vi "main.vi"() -> ()   [LabVIEW 2018]
uses:
  State Enum.ctl
panel:
  in  "Acquisition time":dbl=1.0 caption="Time Target (s)" step=600.0 format="%<%H:%M:%S>t"
  out "Elapsed Time":dbl caption="Elapsed Time (s)" format="%<%H:%M:%S>t"
  in  "Stop":bool
  in  "Time between measurements":dbl=1.0 caption="Time Target (s)" step=10.0 format="%<%H:%M:%S>t"
  out "O3 Reading / V":dbl
  out "O3 Mean / V":dbl format="%0.2f"
  out "NOy Reading / V":dbl
  out "NOy Mean / V":dbl format="%0.2f"
  out "NO2 Reading / V":dbl
  out "NO2 Mean / V":dbl format="%0.2f"
  out "CRDS Voltage":dynamicdata(graph)
  out "NO Reading / V":dbl
  out "NO Mean / V":dbl format="%0.2f"
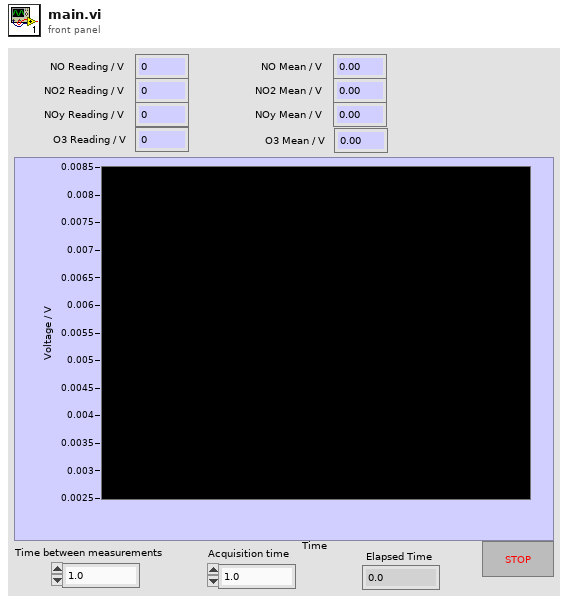
[diagram p1: front panel]
types:
  T1 = enum16{"Always On", "Always Off", "Off While Running"}
  T2 = typedef "State Enum.ctl" = enum16{"Acquisition", "Analysis", "Data Log", "Time Check"}
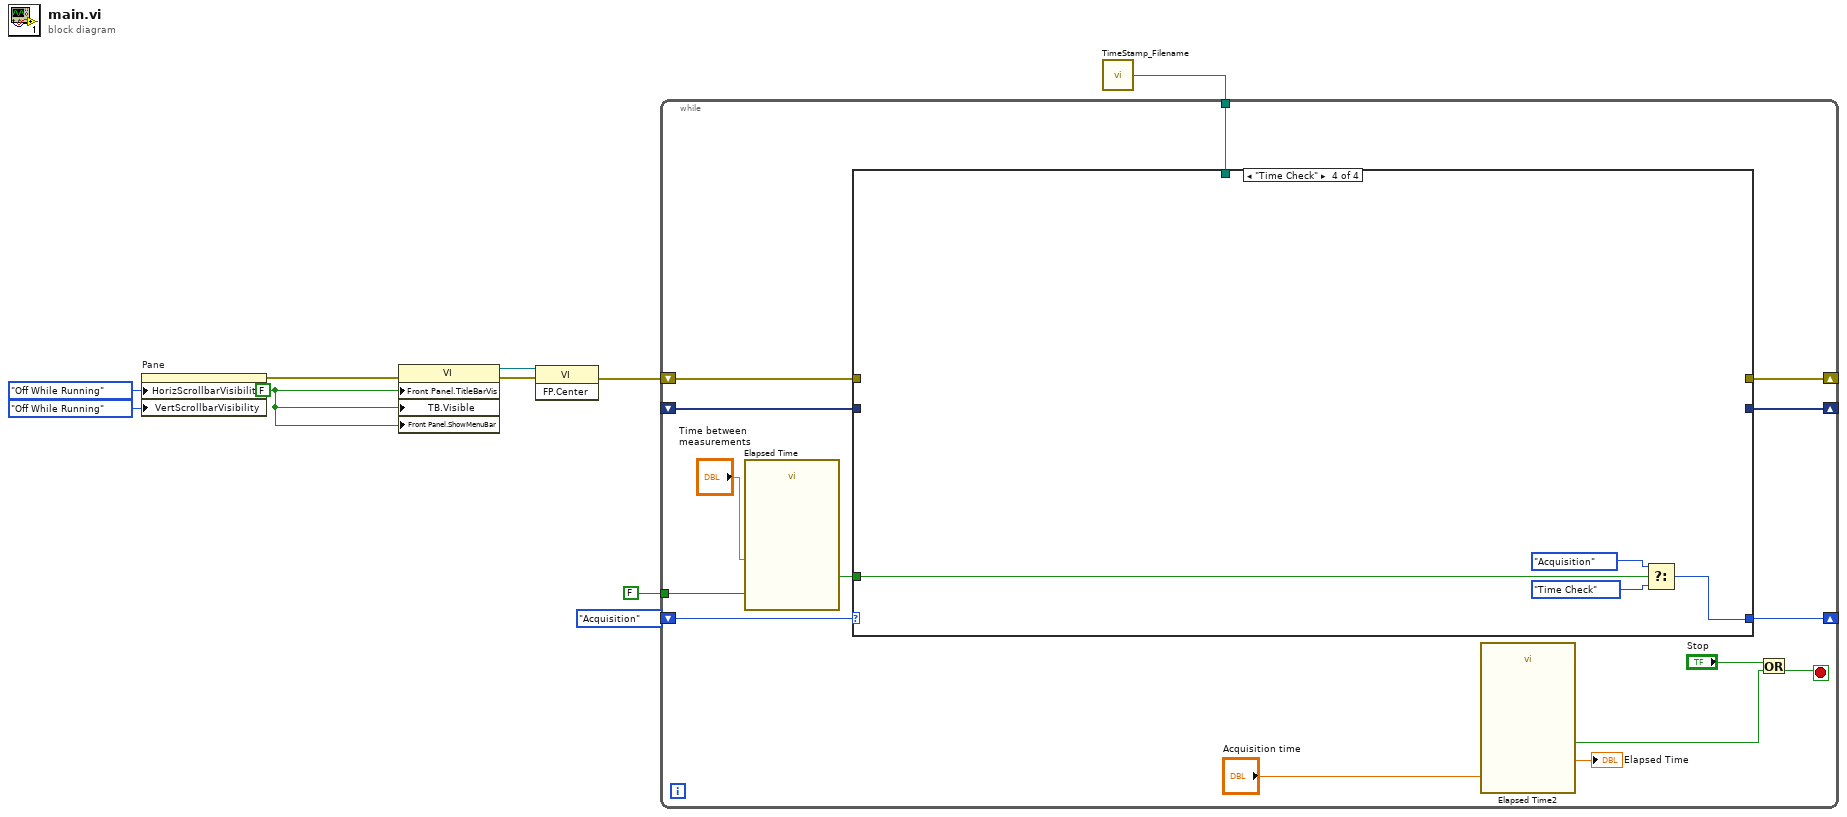
[diagram p0: block diagram]
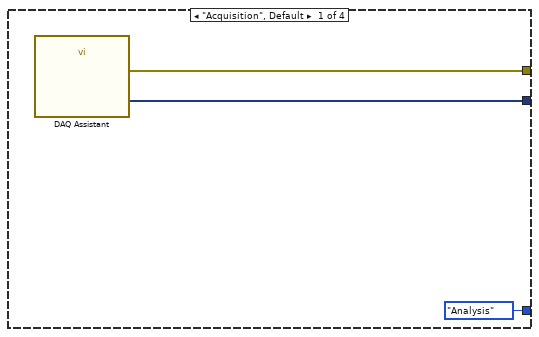
[diagram p2: hidden frame]
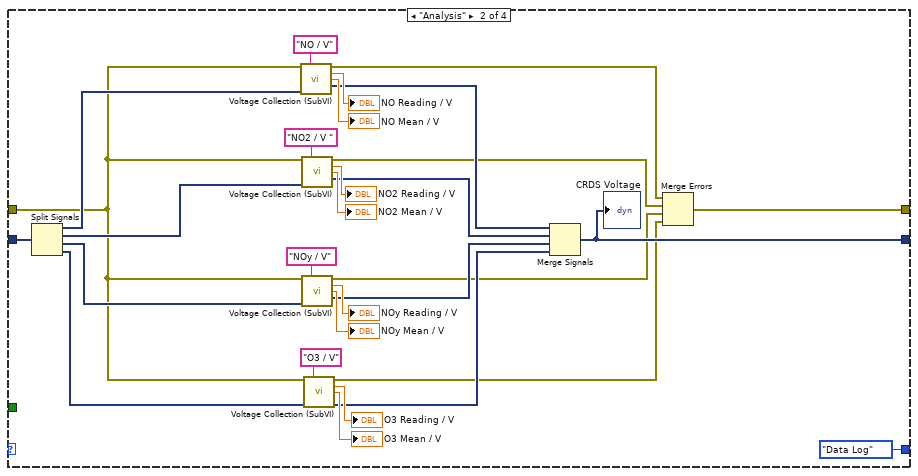
[diagram p3: hidden frame]
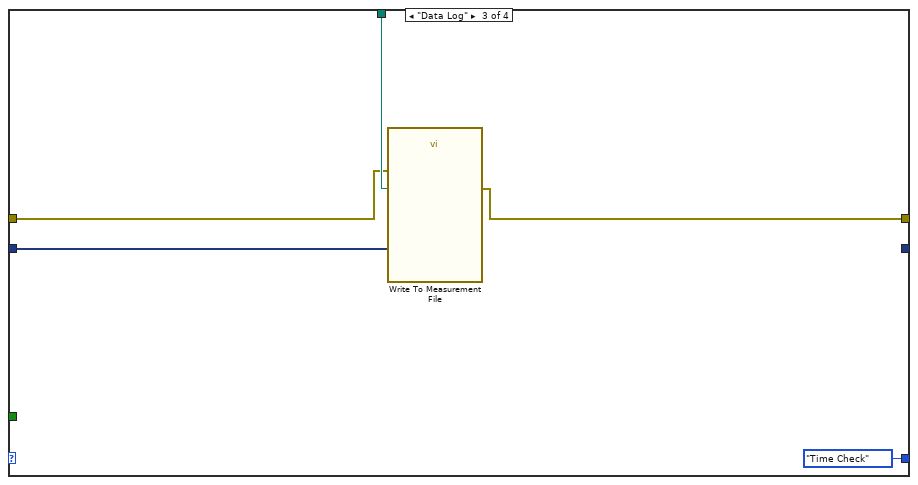
[diagram p4: hidden frame]
diagram:
  w5 = FALSE ("Front Panel Window:Title Bar Visible")
  n1 = property on="Pane" class="Pane"("HorizScrollbarVisibility"=T1."Off While Running" ("Horizontal Scrollbar Visibility"), "VertScrollbarVisibility"=T1."Off While Running" ("Vertical Scrollbar Visibility")) -> (error out=w3:errorcluster)  [unwired: 2 in, 1 out]
  n2 = property class="VI"(error in=w3, "Front Panel.TitleBarVis"=w5, "TB.Visible"=w5, "Front Panel.ShowMenuBar"=w5) -> (reference out=w6:refnum<vi>, error out=w7:errorcluster)  [unwired: 1 in]
  n3 = invoke class="VI" method="FP.Center"(reference=w6, error in=w7) -> (error out=w4:errorcluster)  [unwired: 1 in, 2 out]
  n4 = call "TimeStamp_Filename.vi"() -> ("appended path"=w9:path)
  n5 = while {
    shift-right: [w25] -> _
    shift-left: _ -> [w24]
    shift-right: [w23] -> _
    shift-left: w4 -> [w22]
    tunnel: w9 -> [w20]
    tunnel: FALSE -> [w18]
    shift-right: [w16] -> _
    shift-left: State_Enum."Acquisition" -> [w21]
    stop <- w13 stop-if-true
    n6 = call "Elapsed Time"("Time Target (s)"="Time between measurements", "Reset"=w18) -> ("Time has Elapsed"=w17:bool)  [unwired: 10 in, 7 out]
    n7 = case shown="\"Time Check\"" w21 {
      tunnel: [w28 w35 _ _] -> w25
      tunnel: w24 -> [_ w42 w61 _]
      tunnel: [w27 w34 w59 _] -> w23
      tunnel: w22 -> [_ w37 w60 _]
      tunnel: w20 -> [_ _ w62 _]
      tunnel: w17 -> [_ _ _ w64]
      tunnel: [State_Enum."Analysis" State_Enum."Data Log" State_Enum."Time Check" w63] -> w16
      frame "Acquisition", Default {
        n8 = call "DAQ Assistant"() -> ("data"=w28:dynamicdata, "error out"=w27:errorcluster)  [unwired: 17 in, 1 out]
      }
      frame "Analysis" {
        n9 = Split Signals(w42) -> (w57:dynamicdata, w52:dynamicdata, w49:dynamicdata, w38:dynamicdata)  [unwired: 4 in]
        n10 = call "Voltage Collection (SubVI).vi"("error in (no error)"=w37, "Signal Name"="NO / V", "data"=w57) -> ("error out"=w33:errorcluster, 6:→"NO Reading / V":dbl, 8:→"NO Mean / V":dbl, 10:w53:dynamicdata)  [unwired: 8 in, 1 out]
        n11 = call "Voltage Collection (SubVI).vi"("error in (no error)"=w37, "Signal Name"="NO2 / V ", "data"=w52) -> ("error out"=w32:errorcluster, 6:→"NO2 Reading / V":dbl, 8:→"NO2 Mean / V":dbl, 10:w44:dynamicdata)  [unwired: 8 in, 1 out]
        n12 = call "Voltage Collection (SubVI).vi"("error in (no error)"=w37, "Signal Name"="NOy / V", "data"=w49) -> ("error out"=w31:errorcluster, 6:→"NOy Reading / V":dbl, 8:→"NOy Mean / V":dbl, 10:w43:dynamicdata)  [unwired: 8 in, 1 out]
        n13 = call "Voltage Collection (SubVI).vi"("error in (no error)"=w37, "Signal Name"="O3 / V", "data"=w38) -> ("error out"=w30:errorcluster, 6:→"O3 Reading / V":dbl, 8:→"O3 Mean / V":dbl, "Signals Out"=w36:dynamicdata)  [unwired: 8 in, 1 out]
        n14 = Merge Signals(w53, w44, w43, w36) -> (w35:dynamicdata)
        "CRDS Voltage" <- w35
        n15 = Merge Errors(w33, w32, w31, w30) -> (w34:errorcluster)
      }
      frame "Data Log" {
        n16 = call "Write To Measurement File"("Signals"=w61, "error in (no error)"=w60, "Filename"=w62) -> ("error out"=w59:errorcluster)  [unwired: 14 in, 2 out]
      }
      frame "Time Check" {
        n17 = Select(t=State_Enum."Acquisition", s=w64, f=State_Enum."Time Check") -> (s? t:f=w63:T2)
      }
    }
    n18 = call "Elapsed Time2"("Time Target (s)"="Acquisition time") -> ("Elapsed Time (s)"=→"Elapsed Time":dbl, "Time has Elapsed"=w11:bool)  [unwired: 11 in, 6 out]
    n19 = Or(x="Stop", y=w11) -> (x .or. y?=w13:bool)
  }
